vi "adam5000-run-chassis.vi"(0 "VISA Refnum In":refnum<visa-resource-name>="COM8", 1 "adam-chassis-all-data-in":T9, 3 "adam-chassis-all-DO-in":T7, 4 "adam-chassis-all-AO-in":T3, 5 "error in":errorcluster, 6 "loop-time-in":u32, 7 "adam-chassis-cmd-response-in":T5, 8 "adam-chassis-module-select-in":T2, 9 "adam5000:status-ref-in":T1, 10 "Chassis Settings":T16={"VISA resource name"="COM8", "baud rate (19200)"=19200, "Chassis ID"=1}) -> (12 "loop-time-out":u32, 13 "adam-chassis-cmd-response-out":T5, 14 "VISA Refnum Out":refnum<visa-resource-name>, 15 "adam-chassis-all-data-out":T9, 17 "Loop Time (mS)":u32, 19 "error out":errorcluster)   [LabVIEW 2020]
uses:
  controls/digital-output-cluster.ctl
  controls/digitial-input-cluster.ctl
  controls/analog-input-cluster.ctl
  controls/analog-output-cluster.ctl
  controls/thermocouple-input-cluster.ctl
  controls/adam-5000-all-module-datas.ctl
  controls/adam-5000-all-chassis-data.ctl
  controls/adam-5000-chassis-module-types.ctl
  controls/adam-5000-DO-user-input.ctl
  controls/adam-5000-AO-user-input.ctl
  controls/adam-module-select-tab.ctl
  controls/adam-5000-serial-settings.ctl
  controls/adam-5000-cmd-response.ctl
  controls/adam-5000-chassis-cmd-ack.ctl
  controls/adam-5000-status-indicator-references.ctl
panel:
  out "cmd-response:7":T6
  out "status-indicator:7":cluster{"Sampling":bool, "Ack":bool}
  in  "Slot 7: Module Type":T14(ring)=enum."empty"
  out "slot: 7":T15
  in  "7:Digital Outputs":T8
  out "7:Digital Inputs":T11
  in  "7:Analog Outputs":T4
  out "7:Analog Inputs":T12
  out "7:Thermocouple Inputs (degC)":T13
  out "cmd-response:6":T6
  out "status-indicator:6":cluster{"Sampling":bool, "Ack":bool}
  in  "Slot 6: Module Type":T14(ring)=enum."empty"
  out "slot: 6":T15
  in  "6:Digital Outputs":T8
  out "6:Digital Inputs":T11
  in  "6:Analog Outputs":T4
  out "6:Analog Inputs":T12
  out "6:Thermocouple Inputs (degC)":T13
  out "cmd-response:5":T6
  out "status-indicator:5":cluster{"Sampling":bool, "Ack":bool}
  in  "Slot 5: Module Type":T14(ring)=enum."Analog Output"
  out "slot: 5":T15
  in  "5:Digital Outputs":T8
  out "5:Digital Inputs":T11
  in  "5:Analog Outputs":T4
  out "5:Analog Inputs":T12
  out "5:Thermocouple Inputs (degC)":T13
  out "cmd-response:4":T6
  out "status-indicator:4":cluster{"Sampling":bool, "Ack":bool}
  in  "Slot 4: Module Type":T14(ring)=enum."Power Relay"
  out "slot: 4":T15
  in  "4:Digital Outputs":T8
  out "4:Digital Inputs":T11
  in  "4:Analog Outputs":T4
  out "4:Analog Inputs":T12
  out "4:Thermocouple Inputs (degC)":T13
  out "cmd-response:3":T6
  out "status-indicator:3":cluster{"Sampling":bool, "Ack":bool}
  in  "Slot 3: Module Type":T14(ring)=enum."Thermocouple"
  out "slot: 3":T15
  in  "3:Digital Outputs":T8
  out "3:Digital Inputs":T11
  in  "3:Analog Outputs":T4
  out "3:Analog Inputs":T12
  out "3:Thermocouple Inputs (degC)":T13
  out "cmd-response:2":T6
  out "status-indicator:2":cluster{"Sampling":bool, "Ack":bool}
  in  "Slot 2: Module Type":T14(ring)=enum."Analog Input"
  out "slot: 2":T15
  in  "2:Digital Outputs":T8
  out "2:Digital Inputs":T11
  in  "2:Analog Outputs":T4
  out "2:Analog Inputs":T12
  out "2:Thermocouple Inputs (degC)":T13
  out "cmd-response:1":T6
  out "status-indicator:1":cluster{"Sampling":bool, "Ack":bool}
  in  "Slot 1: Module Type":T14(ring)=enum."Thermocouple"
  out "slot: 1":T15
  in  "1:Digital Outputs":T8
  out "1:Digital Inputs":T11
  in  "1:Analog Outputs":T4
  out "1:Analog Inputs":T12
  out "1:Thermocouple Inputs (degC)":T13
  out "cmd-response:0":T6
  out "status-indicator:0":cluster{"Sampling":bool, "Ack":bool}
  in  "Slot 0: Module Type":T14(ring)=enum."Analog Input"
  out "slot: 0":T15
  in  "0:Digital Outputs":T8
  out "0:Digital Inputs":T11
  in  "0:Analog Outputs":T4
  out "0:Analog Inputs":T12
  out "0:Thermocouple Inputs (degC)":T13
  out "Current Slot":i32
  # "ADAM 5000 Control - SubVI"
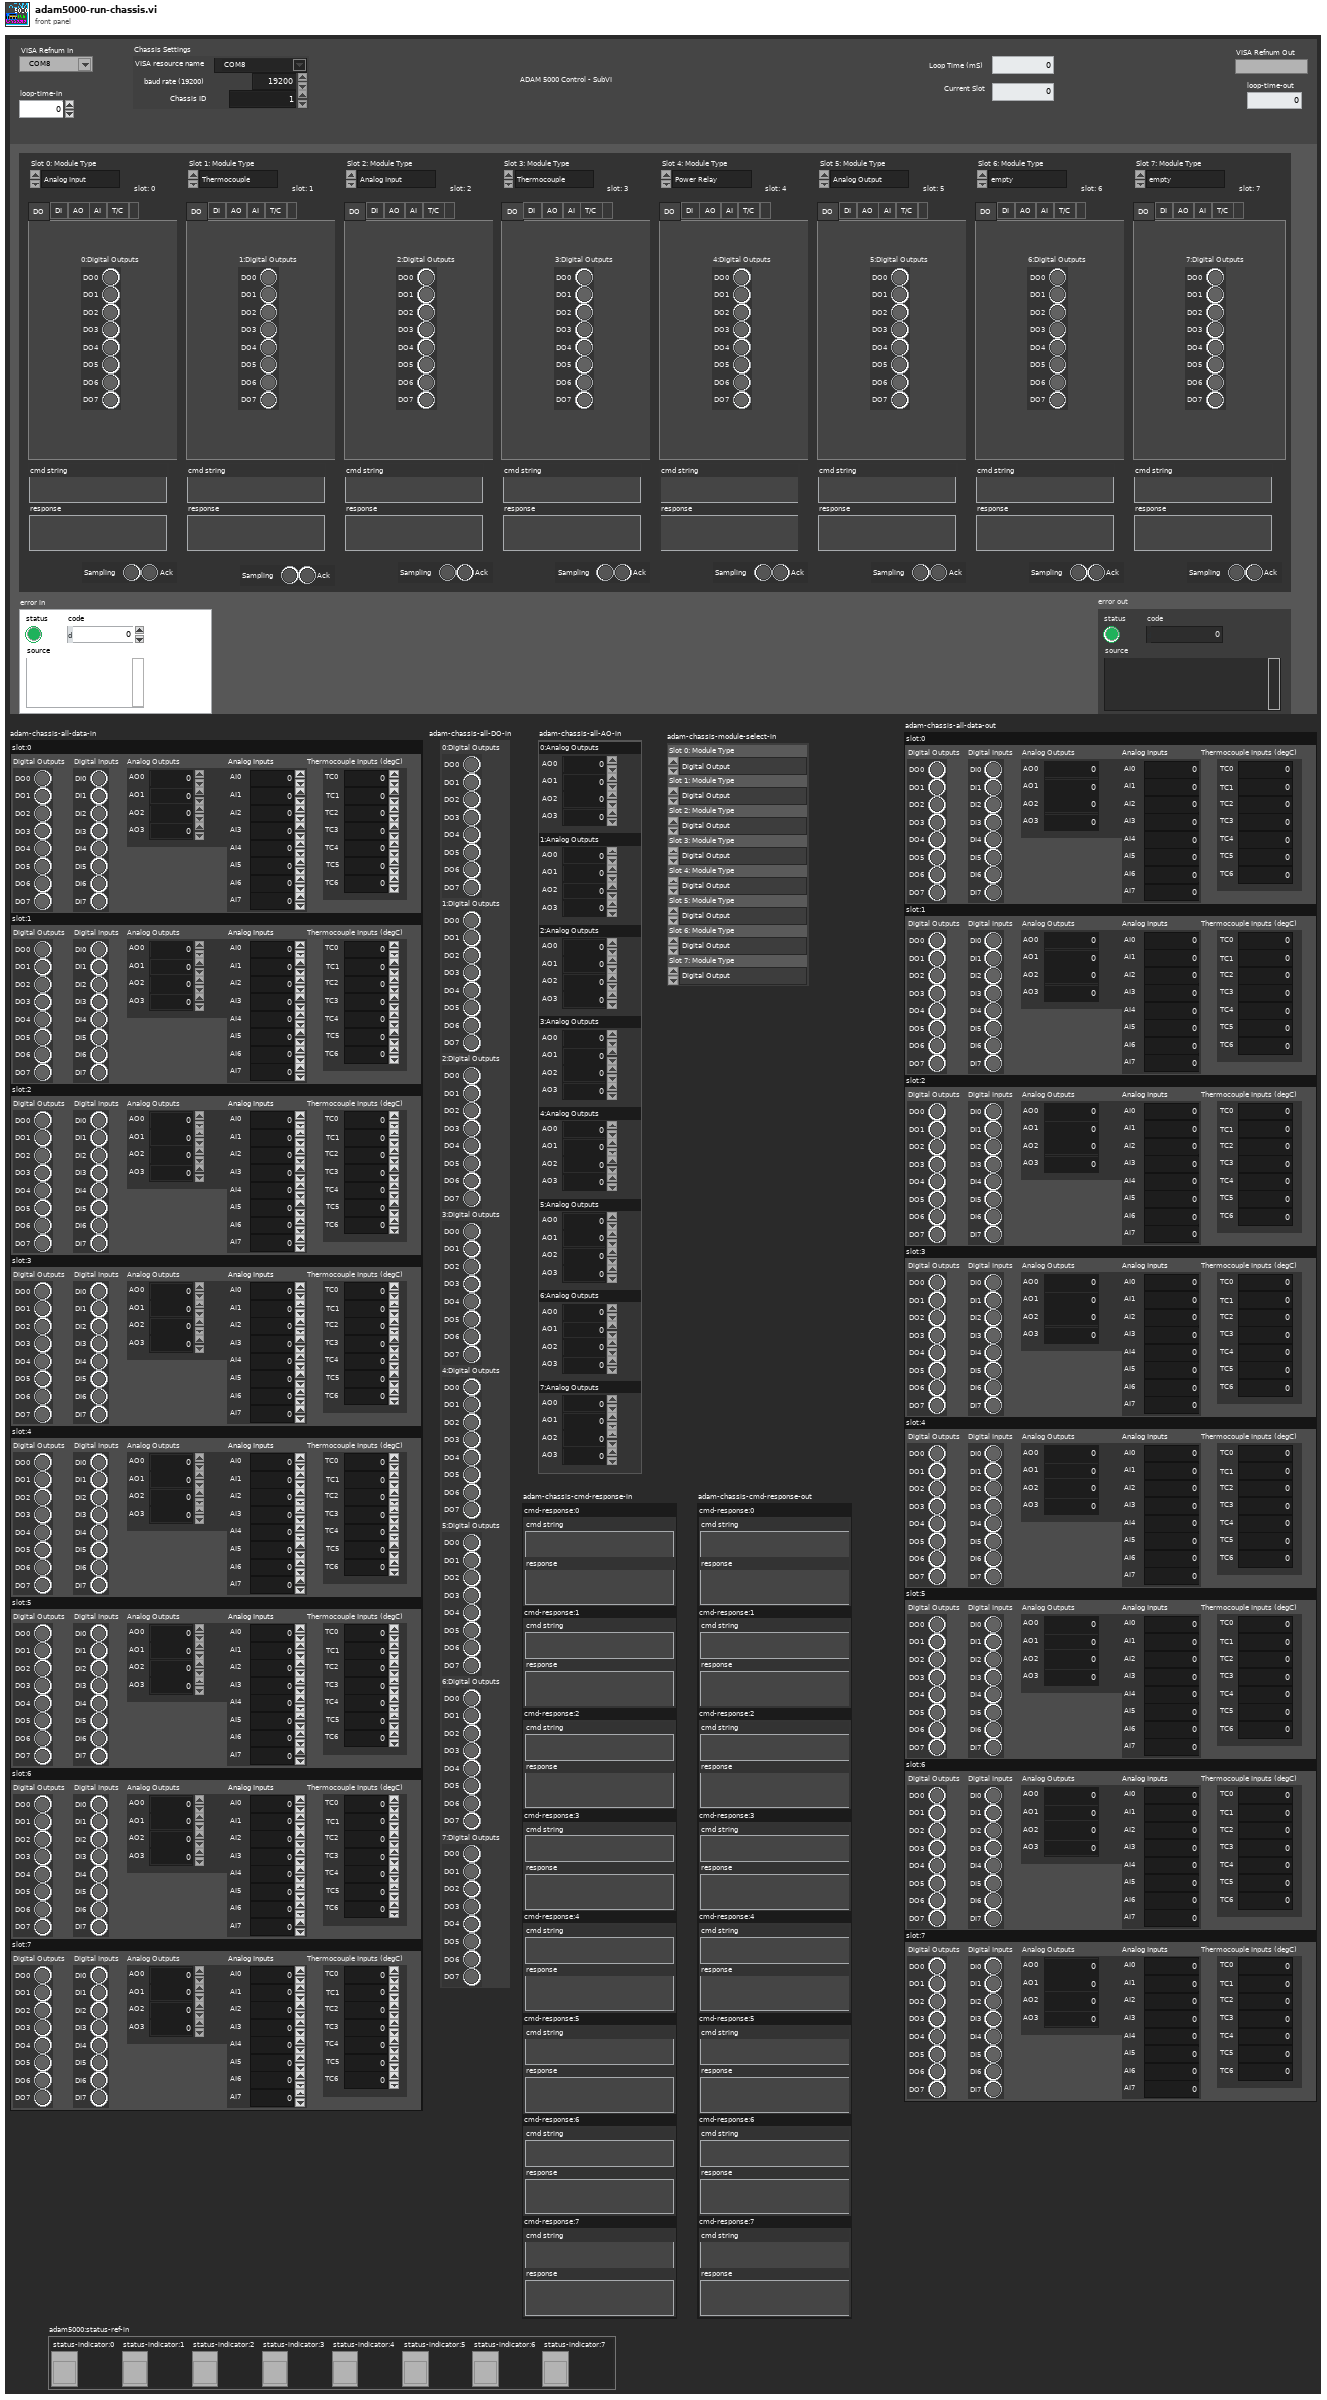
[diagram p1: front panel]
types:
  T1 = typedef "adam-5000-status-indicator-references.ctl" = cluster{"status-indicator:0":refnum<vi>, "status-indicator:1":refnum<vi>, "status-indicator:2":refnum<vi>, "status-indicator:3":refnum<vi>, "status-indicator:4":refnum<vi>, "status-indicator:5":refnum<vi>, "status-indicator:6":refnum<vi>, "status-indicator:7":refnum<vi>}
  T2 = typedef "adam-5000-chassis-module-types.ctl" = cluster{"Slot 0: Module Type":enum16{"Digital Output", "Digital Input", "Analog Output", "Analog Input", "Thermocouple", "Power Relay", "empty"}, "Slot 1: Module Type":enum16{"Digital Output", "Digital Input", "Analog Output", "Analog Input", "Thermocouple", "Power Relay", "empty"}, "Slot 2: Module Type":enum16{"Digital Output", "Digital Input", "Analog Output", "Analog Input", "Thermocouple", "Power Relay", "empty"}, "Slot 3: Module Type":enum16{"Digital Output", "Digital Input", "Analog Output", "Analog Input", "Thermocouple", "Power Relay", "empty"}, "Slot 4: Module Type":enum16{"Digital Output", "Digital Input", "Analog Output", "Analog Input", "Thermocouple", "Power Relay", "empty"}, "Slot 5: Module Type":enum16{"Digital Output", "Digital Input", "Analog Output", "Analog Input", "Thermocouple", "Power Relay", "empty"}, "Slot 6: Module Type":enum16{"Digital Output", "Digital Input", "Analog Output", "Analog Input", "Thermocouple", "Power Relay", "empty"}, "Slot 7: Module Type":enum16{"Digital Output", "Digital Input", "Analog Output", "Analog Input", "Thermocouple", "Power Relay", "empty"}}
  T3 = typedef "adam-5000-AO-user-input.ctl" = cluster{"0:Analog Outputs":T4, "1:Analog Outputs":T4, "2:Analog Outputs":T4, "3:Analog Outputs":T4, "4:Analog Outputs":T4, "5:Analog Outputs":T4, "6:Analog Outputs":T4, "7:Analog Outputs":T4}
  T4 = typedef "analog-output-cluster.ctl" = cluster{"AO0":dbl, "AO1":dbl, "AO2":dbl, "AO3":dbl}
  T5 = typedef "adam-5000-chassis-cmd-ack.ctl" = cluster{"cmd-response:0":T6, "cmd-response:1":T6, "cmd-response:2":T6, "cmd-response:3":T6, "cmd-response:4":T6, "cmd-response:5":T6, "cmd-response:6":T6, "cmd-response:7":T6}
  T6 = typedef "adam-5000-cmd-response.ctl" = cluster{"cmd string":string, "response":string}
  T7 = typedef "adam-5000-DO-user-input.ctl" = cluster{"0:Digital Outputs":T8, "1:Digital Outputs":T8, "2:Digital Outputs":T8, "3:Digital Outputs":T8, "4:Digital Outputs":T8, "5:Digital Outputs":T8, "6:Digital Outputs":T8, "7:Digital Outputs":T8}
  T8 = typedef "digital-output-cluster.ctl" = cluster{"DO0":bool, "DO1":bool, "DO2":bool, "DO3":bool, "DO4":bool, "DO5":bool, "DO6":bool, "DO7":bool}
  T9 = typedef "adam-5000-all-chassis-data.ctl" = cluster{"slot:0":T10, "slot:1":T10, "slot:2":T10, "slot:3":T10, "slot:4":T10, "slot:5":T10, "slot:6":T10, "slot:7":T10}
  T10 = typedef "adam-5000-all-module-datas.ctl" = cluster{"Digital Outputs":T8, "Digital Inputs":T11, "Analog Outputs":T4, "Analog Inputs":T12, "Thermocouple Inputs (degC)":T13}
  T11 = typedef "digitial-input-cluster.ctl" = cluster{"DI0":bool, "DI1":bool, "DI2":bool, "DI3":bool, "DI4":bool, "DI5":bool, "DI6":bool, "DI7":bool}
  T12 = typedef "analog-input-cluster.ctl" = cluster{"AI0":dbl, "AI1":dbl, "AI2":dbl, "AI3":dbl, "AI4":dbl, "AI5":dbl, "AI6":dbl, "AI7":dbl}
  T13 = typedef "thermocouple-input-cluster.ctl" = cluster{"TC0":dbl, "TC1":dbl, "TC2":dbl, "TC3":dbl, "TC4":dbl, "TC5":dbl, "TC6":dbl}
  T14 = enum16{"Digital Output", "Digital Input", "Analog Output", "Analog Input", "Thermocouple", "Power Relay", "empty"}
  T15 = typedef "adam-module-select-tab.ctl" = enum32{"DO", "DI", "AO", "AI", "T/C", ""}
  T16 = typedef "adam-5000-serial-settings.ctl" = cluster{"VISA resource name":refnum<visa-resource-name>, "baud rate (19200)":u32, "Chassis ID":u8}
  T17 = enum16{"Digital Output", "Digital Input", "Analog Output", "Analog Input", "Thermocouple", "Power Relay", "empty"}[]
  T18 = cluster{"[0]":T15, "[1]":T15, "[2]":T15, "[3]":T15, "[4]":T15, "[5]":T15, "[6]":T15, "[7]":T15, "[8]":T15}
  T19 = cluster{"[0]":T10, "[1]":T10, "[2]":T10, "[3]":T10, "[4]":T10, "[5]":T10, "[6]":T10, "[7]":T10, "[8]":T10}
  T20 = cluster{"[0]":T6, "[1]":T6, "[2]":T6, "[3]":T6, "[4]":T6, "[5]":T6, "[6]":T6, "[7]":T6, "[8]":T6}
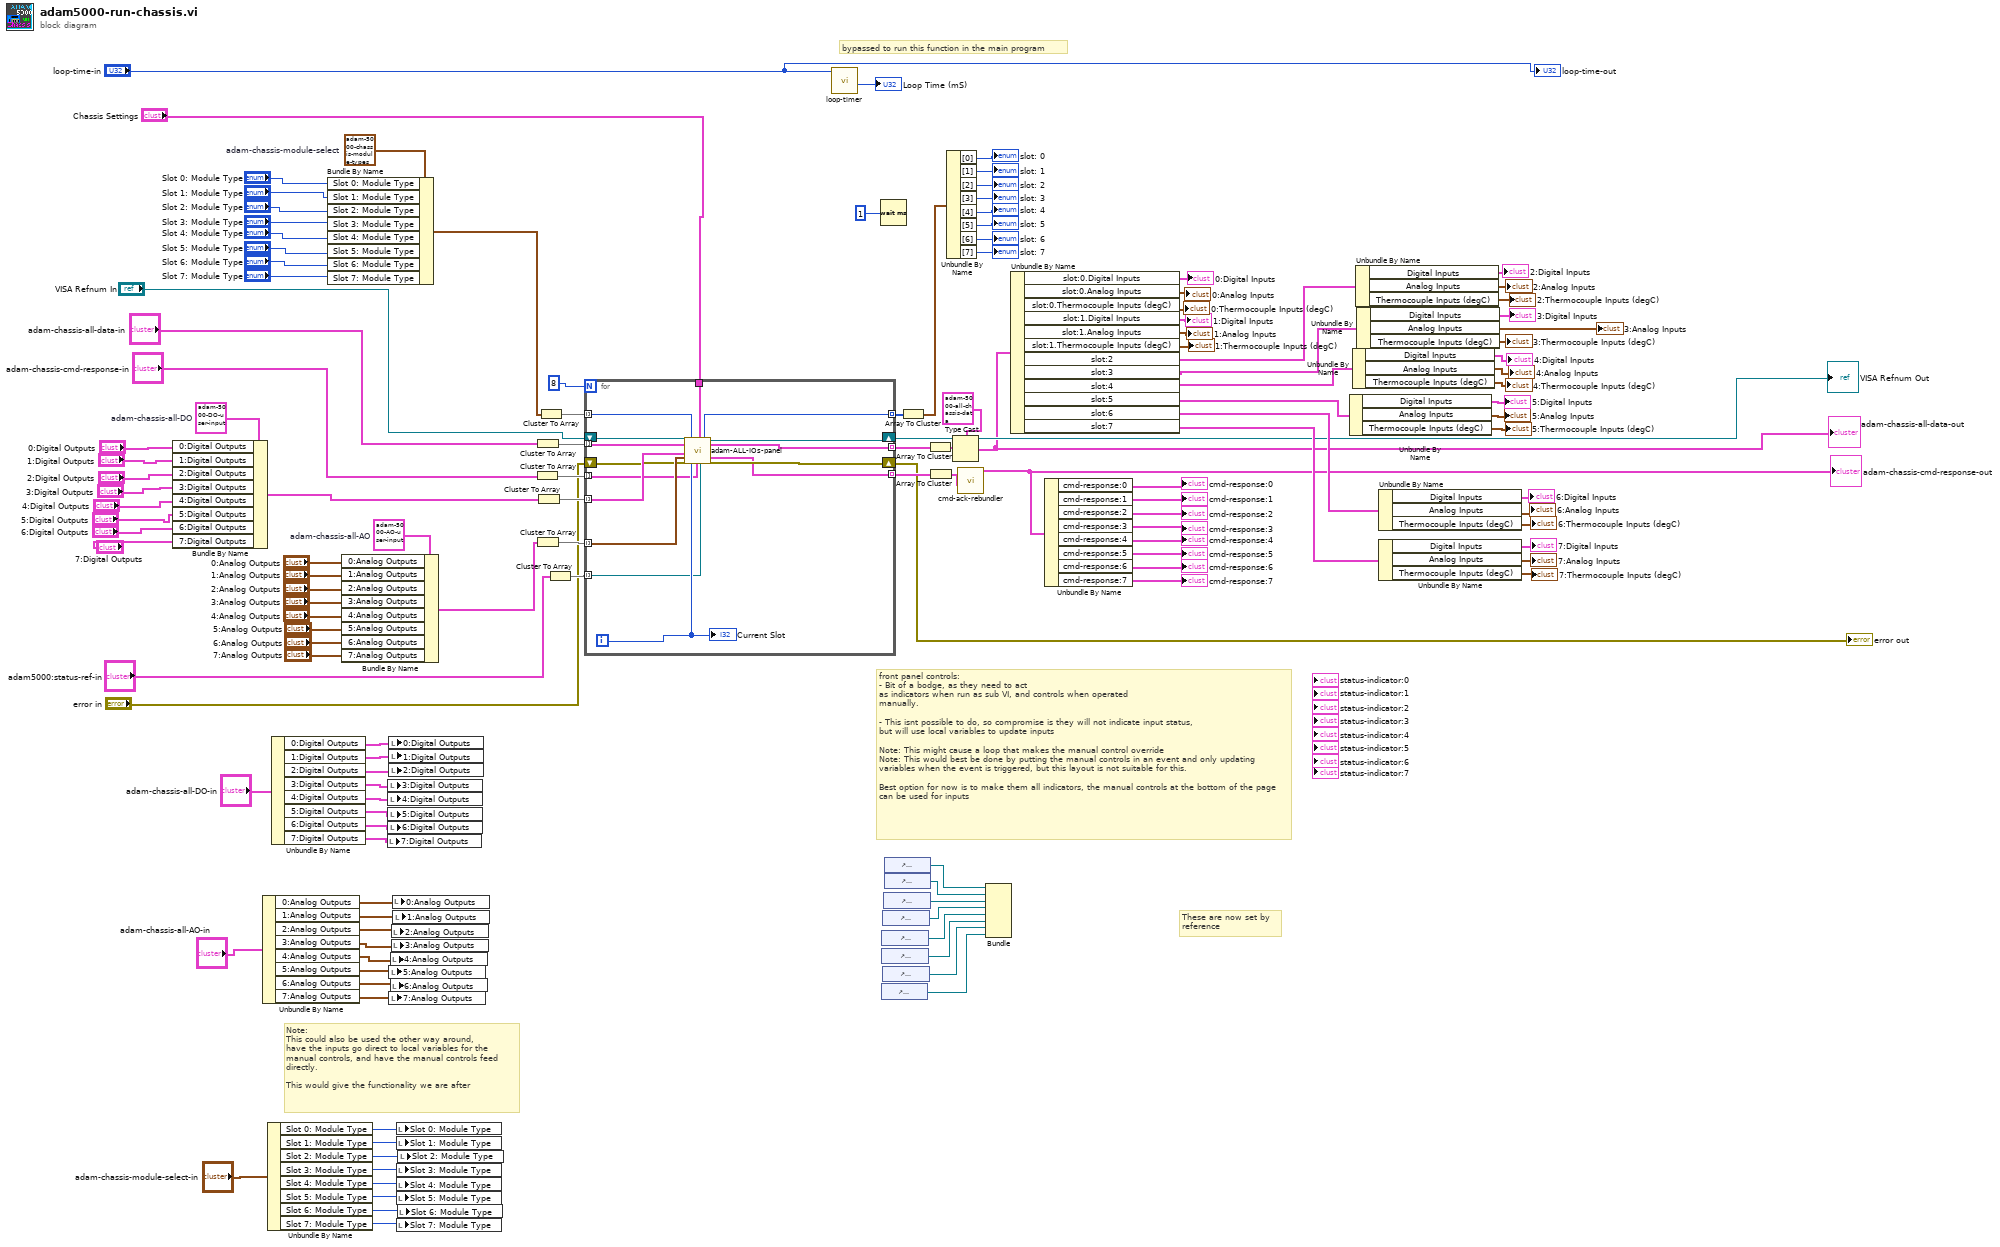
[diagram p0: block diagram]
diagram:
  w45 = T3 {"0:Analog Outputs"={"AO0"=0.0, "AO1"=0.0, "AO2"=0.0, "AO3"=0.0}, "1:Analog Outputs"={"AO0"=0.0, "AO1"=0.0, "AO2"=0.0, "AO3"=0.0}, "2:Analog Outputs"={"AO0"=0.0, "AO1"=0.0, "AO2"=0.0, "AO3"=0.0}, "3:Analog Outputs"={"AO0"=0.0, "AO1"=0.0, "AO2"=0.0, "AO3"=0.0}, "4:Analog Outputs"={"AO0"=0.0, "AO1"=0.0, "AO2"=0.0, "AO3"=0.0}, "5:Analog Outputs"={"AO0"=0.0, "AO1"=0.0, "AO2"=0.0, "AO3"=0.0}, "6:Analog Outputs"={"AO0"=0.0, "AO1"=0.0, "AO2"=0.0, "AO3"=0.0}, "7:Analog Outputs"={"AO0"=0.0, "AO1"=0.0, "AO2"=0.0, "AO3"=0.0}}  # adam-chassis-all-AO
  w44 = T7 {"0:Digital Outputs"={"DO0"=FALSE, "DO1"=FALSE, "DO2"=FALSE, "DO3"=FALSE, "DO4"=FALSE, "DO5"=FALSE, "DO6"=FALSE, "DO7"=FALSE}, "1:Digital Outputs"={"DO0"=FALSE, "DO1"=FALSE, "DO2"=FALSE, "DO3"=FALSE, "DO4"=FALSE, "DO5"=FALSE, "DO6"=FALSE, "DO7"=FALSE}, "2:Digital Outputs"={"DO0"=FALSE, "DO1"=FALSE, "DO2"=FALSE, "DO3"=FALSE, "DO4"=FALSE, "DO5"=FALSE, "DO6"=FALSE, "DO7"=FALSE}, "3:Digital Outputs"={"DO0"=FALSE, "DO1"=FALSE, "DO2"=FALSE, "DO3"=FALSE, "DO4"=FALSE, "DO5"=FALSE, "DO6"=FALSE, "DO7"=FALSE}, "4:Digital Outputs"={"DO0"=FALSE, "DO1"=FALSE, "DO2"=FALSE, "DO3"=FALSE, "DO4"=FALSE, "DO5"=FALSE, "DO6"=FALSE, "DO7"=FALSE}, "5:Digital Outputs"={"DO0"=FALSE, "DO1"=FALSE, "DO2"=FALSE, "DO3"=FALSE, "DO4"=FALSE, "DO5"=FALSE, "DO6"=FALSE, "DO7"=FALSE}, "6:Digital Outputs"={"DO0"=FALSE, "DO1"=FALSE, "DO2"=FALSE, "DO3"=FALSE, "DO4"=FALSE, "DO5"=FALSE, "DO6"=FALSE, "DO7"=FALSE}, "7:Digital Outputs"={"DO0"=FALSE, "DO1"=FALSE, "DO2"=FALSE, "DO3"=FALSE, "DO4"=FALSE, "DO5"=FALSE, "DO6"=FALSE, "DO7"=FALSE}}  # adam-chassis-all-DO
  w43 = T2 {"Slot 0: Module Type"=enum."Digital Output", "Slot 1: Module Type"=enum."Digital Output", "Slot 2: Module Type"=enum."Digital Output", "Slot 3: Module Type"=enum."Digital Output", "Slot 4: Module Type"=enum."Digital Output", "Slot 5: Module Type"=enum."Digital Output", "Slot 6: Module Type"=enum."Digital Output", "Slot 7: Module Type"=enum."Digital Output"}  # adam-chassis-module-select
  # "bypassed to run this function in the main program"
  # "Note:\nThis could also be used the other way around,\nhave the inputs go direct to local variables for the \nmanual controls, and have the manual controls feed\ndirectly. \n\nThis would give the functionality we are after"
  # "front panel controls:\n- Bit of a bodge, as they need to act\nas indicators when run as sub VI, and controls when operated \nmanually.\n\n- This isnt possible to do, so compromise is they will not indicate input status,\nbut will use local variables to update inputs\n\nNote: This might cause a loop that makes the manual control override\nNote: This would best be done by putting the manual controls in an event and only updating\nvariables when the event is triggered, but this layout is not suitable for this.\n\nBest option for now is to make them all indicators, the manual controls at the bottom of the page can be used for inputs"
  # "These are now set by\nreference"
  n1 = Bundle By Name(cluster=w44, "0:Digital Outputs"="0:Digital Outputs", "1:Digital Outputs"="1:Digital Outputs", "2:Digital Outputs"="2:Digital Outputs", "3:Digital Outputs"="3:Digital Outputs", "4:Digital Outputs"="4:Digital Outputs", "5:Digital Outputs"="5:Digital Outputs", "6:Digital Outputs"="6:Digital Outputs", "7:Digital Outputs"="7:Digital Outputs") -> (w5:T7)
  n2 = Unbundle By Name("adam-chassis-all-AO-in") -> ("0:Analog Outputs"=w22:T4, "1:Analog Outputs"=w21:T4, "2:Analog Outputs"=w20:T4, "3:Analog Outputs"=w19:T4, "4:Analog Outputs"=w18:T4, "5:Analog Outputs"=w17:T4, "6:Analog Outputs"=w16:T4, "7:Analog Outputs"=w15:T4)
  n3 = Unbundle By Name("adam-chassis-module-select-in") -> ("Slot 0: Module Type"=w13:T14, "Slot 1: Module Type"=w12:T14, "Slot 2: Module Type"=w11:T14, "Slot 3: Module Type"=w10:T14, "Slot 4: Module Type"=w9:T14, "Slot 5: Module Type"=w8:T14, "Slot 6: Module Type"=w7:T14, "Slot 7: Module Type"=w6:T14)
  n4 = Unbundle By Name("adam-chassis-all-DO-in") -> ("0:Digital Outputs"=w31:T8, "1:Digital Outputs"=w30:T8, "2:Digital Outputs"=w29:T8, "3:Digital Outputs"=w28:T8, "4:Digital Outputs"=w27:T8, "5:Digital Outputs"=w26:T8, "6:Digital Outputs"=w25:T8, "7:Digital Outputs"=w24:T8)
  n5 = Bundle By Name(cluster=w43, "Slot 0: Module Type"="Slot 0: Module Type", "Slot 1: Module Type"="Slot 1: Module Type", "Slot 2: Module Type"="Slot 2: Module Type", "Slot 3: Module Type"="Slot 3: Module Type", "Slot 4: Module Type"="Slot 4: Module Type", "Slot 5: Module Type"="Slot 5: Module Type", "Slot 6: Module Type"="Slot 6: Module Type", "Slot 7: Module Type"="Slot 7: Module Type") -> (w3:T2)
  n6 = Bundle By Name(cluster=w45, "0:Analog Outputs"="0:Analog Outputs", "1:Analog Outputs"="1:Analog Outputs", "2:Analog Outputs"="2:Analog Outputs", "3:Analog Outputs"="3:Analog Outputs", "4:Analog Outputs"="4:Analog Outputs", "5:Analog Outputs"="5:Analog Outputs", "6:Analog Outputs"="6:Analog Outputs", "7:Analog Outputs"="7:Analog Outputs") -> (w4:T3)
  n7 = local write "7:Digital Outputs"(w24) -> ()
  n8 = local write "3:Digital Outputs"(w28) -> ()
  n9 = local write "4:Digital Outputs"(w27) -> ()
  n10 = local write "5:Digital Outputs"(w26) -> ()
  n11 = local write "6:Digital Outputs"(w25) -> ()
  n12 = local write "0:Digital Outputs"(w31) -> ()
  n13 = local write "1:Digital Outputs"(w30) -> ()
  n14 = local write "2:Digital Outputs"(w29) -> ()
  n15 = local write "5:Analog Outputs"(w17) -> ()
  n16 = local write "7:Analog Outputs"(w15) -> ()
  n17 = local write "4:Analog Outputs"(w18) -> ()
  n18 = local write "6:Analog Outputs"(w16) -> ()
  n19 = local write "2:Analog Outputs"(w20) -> ()
  n20 = local write "3:Analog Outputs"(w19) -> ()
  n21 = local write "0:Analog Outputs"(w22) -> ()
  n22 = local write "1:Analog Outputs"(w21) -> ()
  n23 = local write "Slot 0: Module Type"(w13) -> ()
  n24 = local write "Slot 1: Module Type"(w12) -> ()
  n25 = local write "Slot 3: Module Type"(w10) -> ()
  n26 = local write "Slot 4: Module Type"(w9) -> ()
  n27 = local write "Slot 5: Module Type"(w8) -> ()
  n28 = local write "Slot 7: Module Type"(w6) -> ()
  n29 = local write "Slot 6: Module Type"(w7) -> ()
  n30 = local write "Slot 2: Module Type"(w11) -> ()
  n31 = Cluster To Array(cluster="adam-chassis-cmd-response-in") -> (array=w55:T6[])
  n32 = Cluster To Array(cluster="adam-chassis-all-data-in") -> (array=w54:T10[])
  n33 = Cluster To Array(cluster=w4) -> (array=w57:T4[])
  n34 = Cluster To Array(cluster=w5) -> (array=w56:T8[])
  n35 = Cluster To Array(cluster=w3) -> (array=w61:T17)
  n36 = Cluster To Array(cluster="adam5000:status-ref-in") -> (array=w65:refnum<vi>[])
  n37 = for {
    N: 8 -> [_]
    shift-right: [w144] -> w60
    shift-left: "error in" -> [w145]
    shift-right: [w150] -> w37
    shift-left: "VISA Refnum In" -> [w149]
    tunnel: w54 -> [w148] mode=indexing
    tunnel: w55 -> [w140] mode=indexing
    tunnel: w56 -> [w147] mode=indexing
    tunnel: w57 -> [w146] mode=indexing
    tunnel: "Chassis Settings" -> [w152]
    tunnel: w61 -> [w153] mode=indexing
    tunnel: w65 -> [w139] mode=indexing
    tunnel: [w151] -> w66 mode=indexing
    tunnel: [w143] -> w67 mode=indexing
    tunnel: [w142] -> w68 mode=indexing
    i -> [w141]
    n38 = call "adam-ALL-IOs-panel.vi"("VISA Refnum in"=w149, "ADAM-5000-data-current"=w148, "Digital Outputs"=w147, "Analog Outputs"=w146, "error in (no error)"=w145, "Module Type"=w153, "chassis-slot"=w141, "cmd-response in"=w140, "Chassis Settings"=w152, "reference"=w139) -> ("slot: x"=w151:T15, "VISA Refnum out"=w150:refnum<visa-resource-name>, "ADAM-5000-data-new"=w143:T10, "cmd-response out"=w142:T6, "error out"=w144:errorcluster)  [unwired: 5 in]
    "Current Slot" <- w141
  }
  "error out" <- w60
  "VISA Refnum Out" <- w37
  n39 = call "loop-timer.vi"("loop-time-in"="loop-time-in") -> ("Loop Time (mS)"=→"Loop Time (mS)":u32)  [unwired: 8 in, 2 out]
  n40 = Wait (ms)(milliseconds to wait=u32 1) -> ()  [unwired: 1 out]
  n41 = control-ref of="status-indicator:7"() -> (w114:refnum<vi>)
  n42 = control-ref of="status-indicator:4"() -> (w111:refnum<vi>)
  n43 = control-ref of="status-indicator:5"() -> (w112:refnum<vi>)
  n44 = control-ref of="status-indicator:3"() -> (w110:refnum<vi>)
  n45 = control-ref of="status-indicator:6"() -> (w113:refnum<vi>)
  n46 = control-ref of="status-indicator:2"() -> (w80:refnum<vi>)
  n47 = control-ref of="status-indicator:0"() -> (w63:refnum<vi>)
  n48 = control-ref of="status-indicator:1"() -> (w64:refnum<vi>)
  n49 = Array To Cluster(array=w66) -> (cluster=w62:T18)
  n50 = Array To Cluster(array=w67) -> (cluster=w59:T19)
  n51 = Array To Cluster(array=w68) -> (cluster=w75:T20)
  n52 = Unbundle By Name(w62) -> ("[0]"=→"slot: 0":T15, "[1]"=→"slot: 1":T15, "[2]"=→"slot: 2":T15, "[3]"=→"slot: 3":T15, "[4]"=→"slot: 4":T15, "[5]"=→"slot: 5":T15, "[6]"=→"slot: 6":T15, "[7]"=→"slot: 7":T15)
  n53 = Type Cast(type=T9 {"slot:0"={"Digital Outputs"={"DO0"=FALSE, "DO1"=FALSE, "DO2"=FALSE, "DO3"=FALSE, "DO4"=FALSE, "DO5"=FALSE, "DO6"=FALSE, "DO7"=FALSE}, "Digital Inputs"={"DI0"=FALSE, "DI1"=FALSE, "DI2"=FALSE, "DI3"=FALSE, "DI4"=FALSE, "DI5"=FALSE, "DI6"=FALSE, "DI7"=FALSE}, "Analog Outputs"={"AO0"=0.0, "AO1"=0.0, "AO2"=0.0, "AO3"=0.0}, "Analog Inputs"={"AI0"=0.0, "AI1"=0.0, "AI2"=0.0, "AI3"=0.0, "AI4"=0.0, "AI5"=0.0, "AI6"=0.0, "AI7"=0.0}, "Thermocouple Inputs (degC)"={"TC0"=0.0, "TC1"=0.0, "TC2"=0.0, "TC3"=0.0, "TC4"=0.0, "TC5"=0.0, "TC6"=0.0}}, "slot:1"={"Digital Outputs"={"DO0"=FALSE, "DO1"=FALSE, "DO2"=FALSE, "DO3"=FALSE, "DO4"=FALSE, "DO5"=FALSE, "DO6"=FALSE, "DO7"=FALSE}, "Digital Inputs"={"DI0"=FALSE, "DI1"=FALSE, "DI2"=FALSE, "DI3"=FALSE, "DI4"=FALSE, "DI5"=FALSE, "DI6"=FALSE, "DI7"=FALSE}, "Analog Outputs"={"AO0"=0.0, "AO1"=0.0, "AO2"=0.0, "AO3"=0.0}, "Analog Inputs"={"AI0"=0.0, "AI1"=0.0, "AI2"=0.0, "AI3"=0.0, "AI4"=0.0, "AI5"=0.0, "AI6"=0.0, "AI7"=0.0}, "Thermocouple Inputs (degC)"={"TC0"=0.0, "TC1"=0.0, "TC2"=0.0, "TC3"=0.0, "TC4"=0.0, "TC5"=0.0, "TC6"=0.0}}, "slot:2"={"Digital Outputs"={"DO0"=FALSE, "DO1"=FALSE, "DO2"=FALSE, "DO3"=FALSE, "DO4"=FALSE, "DO5"=FALSE, "DO6"=FALSE, "DO7"=FALSE}, "Digital Inputs"={"DI0"=FALSE, "DI1"=FALSE, "DI2"=FALSE, "DI3"=FALSE, "DI4"=FALSE, "DI5"=FALSE, "DI6"=FALSE, "DI7"=FALSE}, "Analog Outputs"={"AO0"=0.0, "AO1"=0.0, "AO2"=0.0, "AO3"=0.0}, "Analog Inputs"={"AI0"=0.0, "AI1"=0.0, "AI2"=0.0, "AI3"=0.0, "AI4"=0.0, "AI5"=0.0, "AI6"=0.0, "AI7"=0.0}, "Thermocouple Inputs (degC)"={"TC0"=0.0, "TC1"=0.0, "TC2"=0.0, "TC3"=0.0, "TC4"=0.0, "TC5"=0.0, "TC6"=0.0}}, "slot:3"={"Digital Outputs"={"DO0"=FALSE, "DO1"=FALSE, "DO2"=FALSE, "DO3"=FALSE, "DO4"=FALSE, "DO5"=FALSE, "DO6"=FALSE, "DO7"=FALSE}, "Digital Inputs"={"DI0"=FALSE, "DI1"=FALSE, "DI2"=FALSE, "DI3"=FALSE, "DI4"=FALSE, "DI5"=FALSE, "DI6"=FALSE, "DI7"=FALSE}, "Analog Outputs"={"AO0"=0.0, "AO1"=0.0, "AO2"=0.0, "AO3"=0.0}, "Analog Inputs"={"AI0"=0.0, "AI1"=0.0, "AI2"=0.0, "AI3"=0.0, "AI4"=0.0, "AI5"=0.0, "AI6"=0.0, "AI7"=0.0}, "Thermocouple Inputs (degC)"={"TC0"=0.0, "TC1"=0.0, "TC2"=0.0, "TC3"=0.0, "TC4"=0.0, "TC5"=0.0, "TC6"=0.0}}, "slot:4"={"Digital Outputs"={"DO0"=FALSE, "DO1"=FALSE, "DO2"=FALSE, "DO3"=FALSE, "DO4"=FALSE, "DO5"=FALSE, "DO6"=FALSE, "DO7"=FALSE}, "Digital Inputs"={"DI0"=FALSE, "DI1"=FALSE, "DI2"=FALSE, "DI3"=FALSE, "DI4"=FALSE, "DI5"=FALSE, "DI6"=FALSE, "DI7"=FALSE}, "Analog Outputs"={"AO0"=0.0, "AO1"=0.0, "AO2"=0.0, "AO3"=0.0}, "Analog Inputs"={"AI0"=0.0, "AI1"=0.0, "AI2"=0.0, "AI3"=0.0, "AI4"=0.0, "AI5"=0.0, "AI6"=0.0, "AI7"=0.0}, "Thermocouple Inputs (degC)"={"TC0"=0.0, "TC1"=0.0, "TC2"=0.0, "TC3"=0.0, "TC4"=0.0, "TC5"=0.0, "TC6"=0.0}}, "slot:5"={"Digital Outputs"={"DO0"=FALSE, "DO1"=FALSE, "DO2"=FALSE, "DO3"=FALSE, "DO4"=FALSE, "DO5"=FALSE, "DO6"=FALSE, "DO7"=FALSE}, "Digital Inputs"={"DI0"=FALSE, "DI1"=FALSE, "DI2"=FALSE, "DI3"=FALSE, "DI4"=FALSE, "DI5"=FALSE, "DI6"=FALSE, "DI7"=FALSE}, "Analog Outputs"={"AO0"=0.0, "AO1"=0.0, "AO2"=0.0, "AO3"=0.0}, "Analog Inputs"={"AI0"=0.0, "AI1"=0.0, "AI2"=0.0, "AI3"=0.0, "AI4"=0.0, "AI5"=0.0, "AI6"=0.0, "AI7"=0.0}, "Thermocouple Inputs (degC)"={"TC0"=0.0, "TC1"=0.0, "TC2"=0.0, "TC3"=0.0, "TC4"=0.0, "TC5"=0.0, "TC6"=0.0}}, "slot:6"={"Digital Outputs"={"DO0"=FALSE, "DO1"=FALSE, "DO2"=FALSE, "DO3"=FALSE, "DO4"=FALSE, "DO5"=FALSE, "DO6"=FALSE, "DO7"=FALSE}, "Digital Inputs"={"DI0"=FALSE, "DI1"=FALSE, "DI2"=FALSE, "DI3"=FALSE, "DI4"=FALSE, "DI5"=FALSE, "DI6"=FALSE, "DI7"=FALSE}, "Analog Outputs"={"AO0"=0.0, "AO1"=0.0, "AO2"=0.0, "AO3"=0.0}, "Analog Inputs"={"AI0"=0.0, "AI1"=0.0, "AI2"=0.0, "AI3"=0.0, "AI4"=0.0, "AI5"=0.0, "AI6"=0.0, "AI7"=0.0}, "Thermocouple Inputs (degC)"={"TC0"=0.0, "TC1"=0.0, "TC2"=0.0, "TC3"=0.0, "TC4"=0.0, "TC5"=0.0, "TC6"=0.0}}, "slot:7"={"Digital Outputs"={"DO0"=FALSE, "DO1"=FALSE, "DO2"=FALSE, "DO3"=FALSE, "DO4"=FALSE, "DO5"=FALSE, "DO6"=FALSE, "DO7"=FALSE}, "Digital Inputs"={"DI0"=FALSE, "DI1"=FALSE, "DI2"=FALSE, "DI3"=FALSE, "DI4"=FALSE, "DI5"=FALSE, "DI6"=FALSE, "DI7"=FALSE}, "Analog Outputs"={"AO0"=0.0, "AO1"=0.0, "AO2"=0.0, "AO3"=0.0}, "Analog Inputs"={"AI0"=0.0, "AI1"=0.0, "AI2"=0.0, "AI3"=0.0, "AI4"=0.0, "AI5"=0.0, "AI6"=0.0, "AI7"=0.0}, "Thermocouple Inputs (degC)"={"TC0"=0.0, "TC1"=0.0, "TC2"=0.0, "TC3"=0.0, "TC4"=0.0, "TC5"=0.0, "TC6"=0.0}}}, x=w59) -> (*(type *) &x=w33:T9)
  "adam-chassis-all-data-out" <- w33
  n54 = call "cmd-ack-rebundler.vi"("cmd-response-in"=w75) -> ("adam-chassis-cmd-response-out"=w74:T5)  [unwired: 10 in]
  "adam-chassis-cmd-response-out" <- w74
  n55 = Bundle("status-indicator:0"=w63, "status-indicator:1"=w64, "status-indicator:2"=w80, "status-indicator:3"=w110, "status-indicator:4"=w111, "status-indicator:5"=w112, "status-indicator:6"=w113, "status-indicator:7"=w114) -> ()  [unwired: 1 in, 1 out]
  n56 = Unbundle By Name(w33) -> ("slot:0.Digital Inputs"=→"0:Digital Inputs":T11, "slot:0.Analog Inputs"=→"0:Analog Inputs":T12, "slot:0.Thermocouple Inputs (degC)"=→"0:Thermocouple Inputs (degC)":T13, "slot:1.Digital Inputs"=→"1:Digital Inputs":T11, "slot:1.Analog Inputs"=→"1:Analog Inputs":T12, "slot:1.Thermocouple Inputs (degC)"=→"1:Thermocouple Inputs (degC)":T13, "slot:2"=w70:T10, "slot:3"=w79:T10, "slot:4"=w85:T10, "slot:5"=w98:T10, "slot:6"=w102:T10, "slot:7"=w103:T10)
  n57 = Unbundle By Name(w74) -> ("cmd-response:0"=→"cmd-response:0":T6, "cmd-response:1"=→"cmd-response:1":T6, "cmd-response:2"=→"cmd-response:2":T6, "cmd-response:3"=→"cmd-response:3":T6, "cmd-response:4"=→"cmd-response:4":T6, "cmd-response:5"=→"cmd-response:5":T6, "cmd-response:6"=→"cmd-response:6":T6, "cmd-response:7"=→"cmd-response:7":T6)
  n58 = Unbundle By Name(w98) -> ("Digital Inputs"=→"5:Digital Inputs":T11, "Analog Inputs"=→"5:Analog Inputs":T12, "Thermocouple Inputs (degC)"=→"5:Thermocouple Inputs (degC)":T13)
  n59 = Unbundle By Name(w85) -> ("Digital Inputs"=→"4:Digital Inputs":T11, "Analog Inputs"=→"4:Analog Inputs":T12, "Thermocouple Inputs (degC)"=→"4:Thermocouple Inputs (degC)":T13)
  n60 = Unbundle By Name(w70) -> ("Digital Inputs"=→"2:Digital Inputs":T11, "Analog Inputs"=→"2:Analog Inputs":T12, "Thermocouple Inputs (degC)"=→"2:Thermocouple Inputs (degC)":T13)
  n61 = Unbundle By Name(w79) -> ("Digital Inputs"=→"3:Digital Inputs":T11, "Analog Inputs"=→"3:Analog Inputs":T12, "Thermocouple Inputs (degC)"=→"3:Thermocouple Inputs (degC)":T13)
  n62 = Unbundle By Name(w102) -> ("Digital Inputs"=→"6:Digital Inputs":T11, "Analog Inputs"=→"6:Analog Inputs":T12, "Thermocouple Inputs (degC)"=→"6:Thermocouple Inputs (degC)":T13)
  n63 = Unbundle By Name(w103) -> ("Digital Inputs"=→"7:Digital Inputs":T11, "Analog Inputs"=→"7:Analog Inputs":T12, "Thermocouple Inputs (degC)"=→"7:Thermocouple Inputs (degC)":T13)
  "loop-time-out" <- "loop-time-in"
